vi "WriteConfiguration.vi"(8 "error in (no error)":errorcluster, 9 "msg body":T10, 10 "body":u8[](array[numeric]), 11 "config":T1={"tcp"=refnum, "ConnInfo"={"ClientName"="", "TransceiverHost"="", "TransceiverPort"=0, "Password"=""}, "SRP"=refnum, "connected"=refnum, "DataSend"={"SendFileMode"=enum."File", "data"=variant, "InProgress"=FALSE}, "Reconnect"={"ReconnectInterval"=0.0, "BaseReconnectInterval"=0.0, "AuthAttempts"=0, "MaxAttempts"=10}, "ProvVersionInfo"={"ConfigurationVersion"="", "ApplicationVersion"="", "ApplicationType"=""}}) -> (0 "error out":errorcluster, 3 "config out":T1={"tcp"=refnum, "ConnInfo"={"ClientName"="", "TransceiverHost"="", "TransceiverPort"=0, "Password"=""}, "SRP"=refnum, "connected"=refnum, "DataSend"={"SendFileMode"=enum."File", "data"=variant, "InProgress"=FALSE}, "Reconnect"={"ReconnectInterval"=0.0, "BaseReconnectInterval"=0.0, "AuthAttempts"=0, "MaxAttempts"=10}, "ProvVersionInfo"={"ConfigurationVersion"="", "ApplicationVersion"="", "ApplicationType"=""}})   [LabVIEW 2017, in "ServerComm.lvlib"]
uses:
  <vilib>/addons/InsightCM/Devices/Shared/Common/ServerComm/ServerComm.lvlib
  <vilib>/addons/InsightCM/MessageBus/MessageLibrary/Device/controls/DeviceConfigurationUpdateRoutedMessageBody.ctl
  <vilib>/addons/InsightCM/MessageBus/Base/controls/DeviceProvisioning.ctl
  <vilib>/addons/InsightCM/MessageBus/Base/controls/DeviceModel.ctl
  <vilib>/addons/InsightCM/MessageBus/Base/controls/Device.ctl
  <vilib>/addons/InsightCM/MessageBus/Base/controls/KeyValuePair.ctl
  <vilib>/addons/InsightCM/MessageBus/Base/controls/DeviceState.ctl
  <vilib>/addons/InsightCM/MessageBus/Base/controls/DataGroup.ctl
  <vilib>/addons/InsightCM/MessageBus/Base/controls/BurstModeTrigger.ctl
  <vilib>/addons/InsightCM/MessageBus/Base/controls/Trigger.ctl
  <vilib>/addons/InsightCM/MessageBus/Base/controls/Condition.ctl
  <vilib>/addons/InsightCM/MessageBus/Base/controls/DeviceSensorGroup.ctl
  <vilib>/addons/InsightCM/MessageBus/Base/controls/WirelessEndpoint.ctl
  <vilib>/addons/InsightCM/MessageBus/Base/controls/WirelessChannel.ctl
  <vilib>/addons/InsightCM/MessageBus/Base/controls/Channel.ctl
  <vilib>/addons/InsightCM/MessageBus/Base/controls/Tag.ctl
  <vilib>/addons/InsightCM/Devices/Shared/Common/ServerComm/controls/config.ctl
  <vilib>/addons/InsightCM/MessageBus/TcpApi/controls/TcpMessageReference.ctl
  <vilib>/addons/InsightCM/MessageBus/Base/controls/ConnectionInfo.ctl
  <vilib>/addons/InsightCM/SRP/controls/DVR_data.ctl
  <vilib>/addons/InsightCM/SRP/controls/data.ctl
  <vilib>/addons/InsightCM/Devices/Shared/Common/ServerComm/controls/ConnectedStatusDvr.ctl
  <vilib>/addons/InsightCM/Devices/Shared/Common/ServerComm/controls/ConnectionStatus.ctl
  <vilib>/addons/InsightCM/Devices/Shared/Common/ServerComm/controls/DataSendStatus.ctl
  <vilib>/addons/InsightCM/Devices/Shared/Common/ServerComm/controls/DataSendMode.ctl
  <vilib>/addons/InsightCM/Devices/Shared/Common/ServerComm/controls/ReconnectData.ctl
  <vilib>/addons/InsightCM/Devices/Shared/Common/ServerComm/controls/ProvisioningVersionInfo.ctl
  <vilib>/addons/InsightCM/SRP/SRP.lvlib
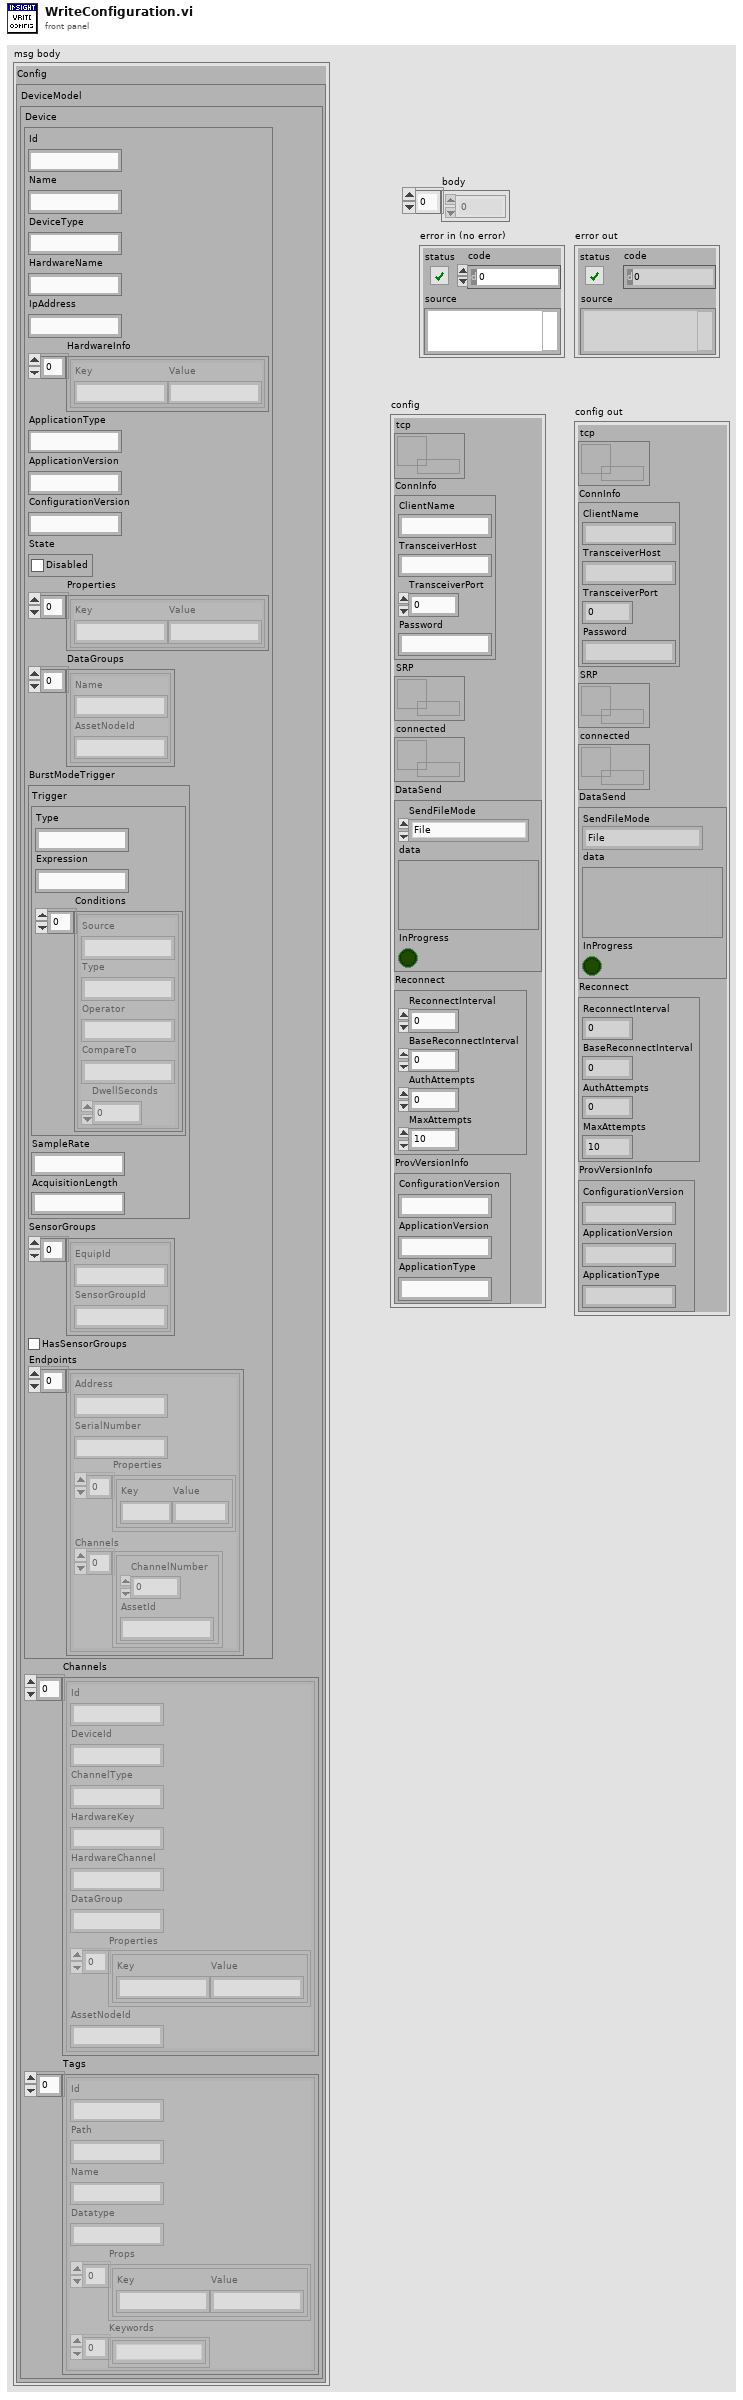
[diagram p1: front panel]
types:
  T1 = typedef "ServerComm.lvlib/config.ctl" = cluster{"tcp":T2, "ConnInfo":T3, "SRP":T4, "connected":T5, "DataSend":T6, "Reconnect":T8, "ProvVersionInfo":T9}
  T2 = typedef "TcpMessageReference.ctl" = refnum<data-value>
  T3 = typedef "ConnectionInfo.ctl" = cluster{"ClientName":string, "TransceiverHost":string, "TransceiverPort":u16, "Password":string}
  T4 = typedef "SRP.lvlib/DVR_data.ctl" = refnum<data-value>
  T5 = typedef "ServerComm.lvlib/ConnectedStatusDvr.ctl" = refnum<data-value>
  T6 = typedef "ServerComm.lvlib/DataSendStatus.ctl" = cluster{"SendFileMode":T7, "data":variant, "InProgress":bool}
  T7 = typedef "ServerComm.lvlib/DataSendMode.ctl" = enum16{"File", "InMemoryFile", "Stream", "StreamFileBlock", "ByteArray", "NoOp", "UnknownData"}
  T8 = typedef "ServerComm.lvlib/ReconnectData.ctl" = cluster{"ReconnectInterval":dbl, "BaseReconnectInterval":dbl, "AuthAttempts":i32, "MaxAttempts":i32}
  T9 = typedef "ServerComm.lvlib/ProvisioningVersionInfo.ctl" = cluster{"ConfigurationVersion":string, "ApplicationVersion":string, "ApplicationType":string}
  T10 = typedef "DeviceConfigurationUpdateRoutedMessageBody.ctl" = cluster{"Config":T11}
  T11 = typedef "DeviceProvisioning.ctl" = cluster{"DeviceModel":T12}
  T12 = typedef "DeviceModel.ctl" = cluster{"Device":T13, "Channels":T23[], "Tags":T24[]}
  T13 = typedef "Device.ctl" = cluster{"Id":string, "Name":string, "DeviceType":string, "HardwareName":string, "IpAddress":string, "HardwareInfo":T14[], "ApplicationType":string, "ApplicationVersion":string, "ConfigurationVersion":string, "State":T15, "Properties":T14[], "DataGroups":T16[], "BurstModeTrigger":T17, "SensorGroups":T20[], "HasSensorGroups":bool, "Endpoints":T21[]}
  T14 = typedef "KeyValuePair.ctl" = cluster{"Key":string, "Value":string}
  T15 = typedef "DeviceState.ctl" = cluster{"Disabled":bool}
  T16 = typedef "DataGroup.ctl" = cluster{"Name":string, "AssetNodeId":string}
  T17 = typedef "BurstModeTrigger.ctl" = cluster{"Trigger":T18, "SampleRate":string, "AcquisitionLength":string}
  T18 = typedef "Trigger.ctl" = cluster{"Type":string, "Expression":string, "Conditions":T19[]}
  T19 = typedef "Condition.ctl" = cluster{"Source":string, "Type":string, "Operator":string, "CompareTo":string, "DwellSeconds":dbl}
  T20 = typedef "DeviceSensorGroup.ctl" = cluster{"EquipId":string, "SensorGroupId":string}
  T21 = typedef "WirelessEndpoint.ctl" = cluster{"Address":string, "SerialNumber":string, "Properties":T14[], "Channels":T22[]}
  T22 = typedef "WirelessChannel.ctl" = cluster{"ChannelNumber":i32, "AssetId":string}
  T23 = typedef "Channel.ctl" = cluster{"Id":string, "DeviceId":string, "ChannelType":string, "HardwareKey":string, "HardwareChannel":string, "DataGroup":string, "Properties":T14[], "AssetNodeId":string}
  T24 = typedef "Tag.ctl" = cluster{"Id":string, "Path":string, "Name":string, "Datatype":string, "Props":T14[], "Keywords":string[]}
  T25 = typedef "R2_DeviceModel.ctl" = cluster{"Device":T26, "Channels":T29[], "Tags":T24[]}
  T26 = typedef "R2_Device.ctl" = cluster{"Id":string, "Name":string, "DeviceType":string, "HardwareName":string, "IpAddress":string, "HardwareInfo":T14[], "ApplicationType":string, "ApplicationVersion":string, "EquipmentIds":string[], "ConfigurationVersion":string, "State":T15, "Properties":T14[], "DataGroups":T27[], "BurstModeTrigger":T17, "SensorGroups":T20[], "Endpoints":T21[]}
  T27 = typedef "R2_DataGroup.ctl" = cluster{"Name":string, "OperatingStates":T28[], "Properties":T14[], "EquipmentIds":string[], "AssetNodeId":string}
  T28 = typedef "OperatingState.ctl" = cluster{"Name":string, "Properties":T14[], "Triggers":T18[]}
  T29 = typedef "R2_Channel.ctl" = cluster{"Id":string, "DeviceId":string, "Name":string, "ChannelType":string, "HardwareKey":string, "HardwareChannel":string, "DataGroup":string, "Keywords":string[], "EquipmentIds":string[], "Properties":T14[], "Metrics":T30[], "AssetNodeId":string, "MeasType":string, "AssetName":string}
  T30 = typedef "Metric.ctl" = cluster{"Id":string, "Name":string, "Unit":string, "Properties":T14[], "MetricDefinitionInstanceId":string}
  T31 = typedef "AssetNode.ctl" = cluster{"Id":string, "Type":string, "Name":string, "ParentIds":string[], "State":T32, "MeasType":string, "Properties":T14[], "SensorGroups":T33[], "OperatingStates":T28[], "Metrics":T30[], "TrendAlarmRules":T34[], "References":T37[]}
  T32 = typedef "AssetState.ctl" = cluster{"Disabled":bool}
  T33 = typedef "AssetNodeSensorGroup.ctl" = cluster{"Id":string, "Type":string, "SensorIds":string[], "Triggers":T18[], "Properties":T14[]}
  T34 = typedef "TrendAlarmRule.ctl" = cluster{"Id":string, "AssetNodeId":string, "TrendId":string, "Disabled":bool, "OperatingState":string, "Operator":string, "Hysteresis":dbl, "OnDelaySeconds":dbl, "OffDelaySeconds":dbl, "Levels":T35[], "Properties":T14[]}
  T35 = typedef "TrendAlarmLevel.ctl" = cluster{"Severity":i32, "CompareTo":dbl, "Actions":T36[]}
  T36 = typedef "AlarmAction.ctl" = cluster{"Type":string, "Props":T14[]}
  T37 = typedef "AssetNodeReference.ctl" = cluster{"NodeId":string, "Name":string}
  T38 = typedef "SectionKeyValues.ctl" = cluster{"Section":string, "KeyValues":T14[]}
  T39 = typedef "Camera.ctl" = cluster{"Id":string, "Name":string, "Properties":T14[], "Triggers":T18[]}
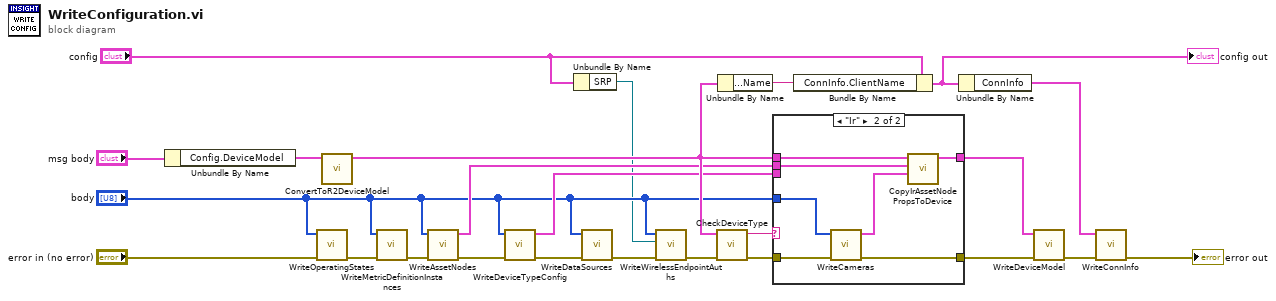
[diagram p0: block diagram]
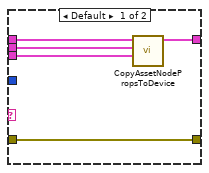
[diagram p2: hidden frame]
diagram:
  n1 = Unbundle By Name("msg body") -> ("Config.DeviceModel"=w18:T12)
  n2 = call <vilib>:"WriteOperatingStates.vi"("error in (no error)"="error in (no error)", "body"="body") -> ("error out"=w14:errorcluster)  [unwired: 9 in]
  n3 = call <vilib>:"ConvertToR2DeviceModel.vi"("DeviceModel"=w18) -> ("R2 DeviceModel"=w17:T25)  [unwired: 10 in]
  n4 = call <vilib>:"WriteMetricDefinitionInstances.vi"("error in (no error)"=w14, "body"="body") -> ("error out"=w11:errorcluster)  [unwired: 9 in]
  n5 = call <vilib>:"WriteAssetNodes.vi"("error in (no error)"=w11, "body"="body") -> ("error out"=w10:errorcluster, "asset nodes"=w16:T31[])  [unwired: 8 in]
  n6 = call <vilib>:"WriteDeviceTypeConfig.vi"("error in (no error)"=w10, "body"="body") -> ("error out"=w7:errorcluster, "key values"=w12:T38[])  [unwired: 8 in]
  n7 = Unbundle By Name("config") -> ("SRP"=w1:T4)
  n8 = call <vilib>:"WriteDataSources.vi"("error in (no error)"=w7, "body"="body") -> ("error out"=w8:errorcluster)  [unwired: 9 in]
  n9 = call <vilib>:"WriteWirelessEndpointAuths.vi"("error in (no error)"=w8, "SRP"=w1, "body"="body") -> ("error out"=w6:errorcluster)  [unwired: 8 in]
  n10 = call <vilib>:"CheckDeviceType.vi"("error in (no error)"=w6, "R2 DeviceModel"=w17) -> ("error out"=w21:errorcluster, "device"=w20:string)  [unwired: 8 in]
  n11 = Unbundle By Name(w17) -> ("Device.Name"=w5:string)
  n12 = case shown="\"Ir\"" w20 {
    tunnel: [w29 w36] -> w23
    tunnel: [w25 w34] -> w13
    tunnel: w21 -> [w25 w35]
    tunnel: "body" -> [_ w32]
    tunnel: w17 -> [w28 w33]
    tunnel: w16 -> [w27 w30]
    tunnel: w12 -> [w26 _]
    frame Default {
      n13 = call <vilib>:"CopyAssetNodePropsToDevice.vi"("KeyValues"=w26, "AssetNodes"=w27, "DeviceModel in"=w28) -> ("DeviceModel out"=w29:T25)  [unwired: 8 in]
    }
    frame "Ir" {
      n14 = call <vilib>:"WriteCameras.vi"("error in (no error)"=w35, "body"=w32) -> ("error out"=w34:errorcluster, "cameras"=w31:T39[])  [unwired: 8 in]
      n15 = call <vilib>:"CopyIrAssetNodePropsToDevice.vi"("Cameras"=w31, "AssetNodes"=w30, "DeviceModel in"=w33) -> ("DeviceModel out"=w36:T25)  [unwired: 8 in]
    }
  }
  n16 = Bundle By Name(cluster="config", "ConnInfo.ClientName"=w5) -> (w4:T1)
  "config out" <- w4
  n17 = Unbundle By Name(w4) -> ("ConnInfo"=w3:T3)
  n18 = call <vilib>:"WriteDeviceModel.vi"("error in (no error)"=w13, "device model"=w23) -> ("error out"=w22:errorcluster)  [unwired: 9 in]
  n19 = call <vilib>:"WriteConnInfo.vi"("error in (no error)"=w22, "connection info"=w3) -> ("error out"=→"error out":errorcluster)  [unwired: 9 in]
